vi "Untitled 3.vi"() -> ()   [LabVIEW 2013]
panel:
  out "size(*)":i32
  out "size(B)":i32
  out "size(A)":i32
  out "x*y":dbl[](array[numeric])
  in  "B":dbl[](array[numeric])
  in  "A":dbl[](array[numeric])
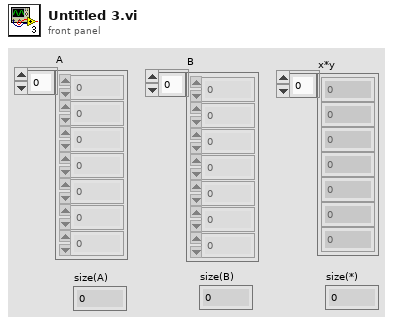
[diagram p1: front panel]
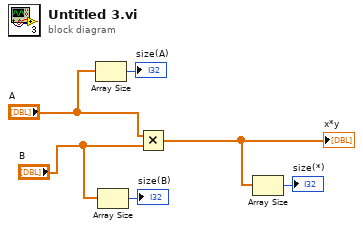
[diagram p0: block diagram]
diagram:
  n1 = Array Size(array="A") -> (size(s)=→"size(A)":i32)
  n2 = Array Size(array="B") -> (size(s)=→"size(B)":i32)
  n3 = Multiply(x="A", y="B") -> (x*y=w1:dbl[])
  "x*y" <- w1
  n4 = Array Size(array=w1) -> (size(s)=→"size(*)":i32)
